vi "CursorSet.vi"(8 "错误输入":errorcluster caption="错误输入（无错误）", 11 "WG":refnum<vi>) -> (0 "错误输出":errorcluster, 2 "MIN":dbl, 3 "MAX":dbl)   [LabVIEW 2012]
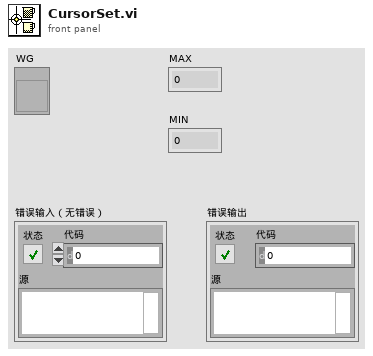
[diagram p1: front panel]
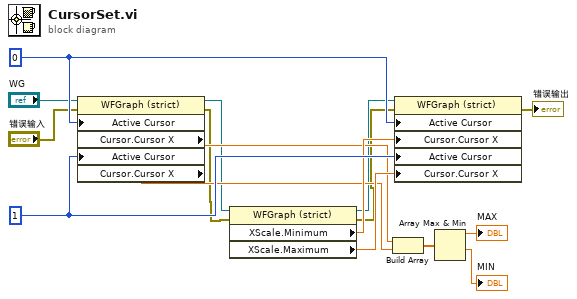
[diagram p0: block diagram]
diagram:
  w16 = u32 1 ("活动游标")
  w13 = u32 0 ("活动游标")
  n1 = property on="属性节点" class="WFGraph (strict)"(reference="WG", error in="错误输入", "Active Cursor"=w13, "Active Cursor"=w16) -> (reference out=w4:refnum<vi>, error out=w1:errorcluster, "Cursor.Cursor X"=w8:dbl, "Cursor.Cursor X"=w9:dbl)
  n2 = property on="属性节点" class="WFGraph (strict)"(reference=w4, error in=w1) -> (reference out=w3:refnum<vi>, error out=w2:errorcluster, "XScale.Minimum"=w14:dbl, "XScale.Maximum"=w15:dbl)
  n3 = Build Array(w8, w9) -> (w10:dbl[])
  n4 = property on="属性节点" class="WFGraph (strict)"(reference=w3, error in=w2, "Active Cursor"=w13, "Cursor.Cursor X"=w14, "Active Cursor"=w16, "Cursor.Cursor X"=w15) -> (error out=→"错误输出":errorcluster)  [unwired: 1 out]
  n5 = Array Max & Min(array=w10) -> (max value=→"MAX":dbl, min value=→"MIN":dbl)  [unwired: 2 out]
